vi "Indefinite Integral of Polynomial (CDB).vi"(11 "P(x)":cdb[](array[numeric])) -> (0 "error":i32, 3 "Indefinite Integral of P(x)":cdb[](array[numeric]))   [LabVIEW 2020, in "NI_AALPro.lvlib"]
doc: "Calculates the indefinite integral of <B>P(x)</B>. Wire data to the <B>P(x)</B> input to determine the polymorphic instance to use or manually select the instance."
uses:
  <vilib>/Analysis/NI_AALPro.lvlib
  <vilib>/Analysis/1siggen.llb/Ramp Pattern by Samples.vi
  <vilib>/Analysis/NI_AALBase.lvlib
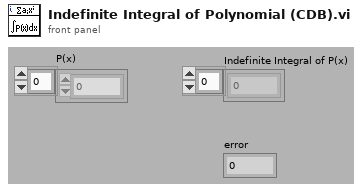
[diagram p1: front panel]
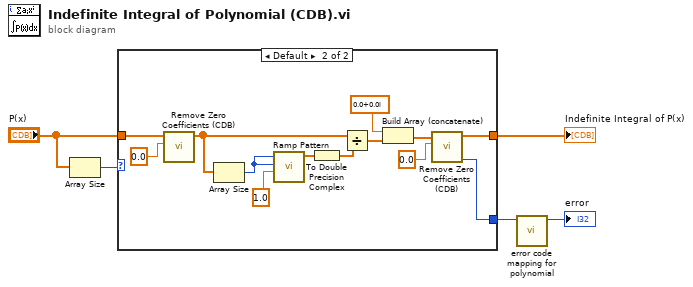
[diagram p0: block diagram]
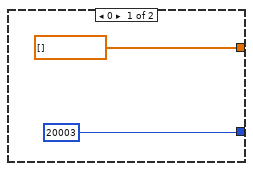
[diagram p2: hidden frame]
diagram:
  n1 = Array Size(array="P(x)") -> (size(s)=w4:i32)
  n2 = case shown="Default" w4 {
    tunnel: [cdb[] [] ("CDB") w15] -> w3
    tunnel: "P(x)" -> [_ w19]
    tunnel: [20003 ("empty array") w14] -> w2
    frame 0 {
    }
    frame Default {
      n3 = call <vilib>:"Remove Zero Coefficients (CDB).vi"("threshold"=0.0, "P(x) In"=w19) -> ("P(x) Out"=w9:cdb[])  [unwired: 7 in, 2 out]
      n4 = Array Size(array=w9) -> (size(s)=w13:i32)
      n5 = call-poly <vilib>:"Ramp Pattern.vi"("start"=1.0, "end"=w13, "samples"=w13) -> ("Ramp Pattern"=w11:dbl[])  [unwired: 7 in, 1 out]
      n6 = To Double Precision Complex(1:w11) -> (0:w10:cdb[])
      n7 = Divide(x=w9, y=w10) -> (x/y=w8:cdb[])
      n8 = Build Array (concatenate)(cdb 0.0+0.0i, w8) -> (w16:cdb[])
      n9 = call <vilib>:"Remove Zero Coefficients (CDB).vi"("threshold"=0.0, "P(x) In"=w16) -> ("error"=w14:i32, "P(x) Out"=w15:cdb[])  [unwired: 7 in, 1 out]
    }
  }
  "Indefinite Integral of P(x)" <- w3
  n10 = call <vilib>:"error code mapping for polynomial.vi"("error in"=w2) -> ("error out"=→"error":i32)  [unwired: 10 in]
